vi "Get nidaqmx_grpc_GetChanAttributeStringRequest.vi"(8 "error in (no error)":errorcluster, 11 "gRPCid":T1) -> (0 "error out":errorcluster, 2 "package_templatemessage":T2, 3 "gRPCid out":T1)   [LabVIEW 2021, in "NI DAQmx_server.lvlib"]
uses:
  NI DAQmx_server.lvlib
  nidaqmx_grpc_GetChanAttributeStringRequest.ctl
  nidevice_grpc_Session_session/nidevice_grpc_Session_session.lvclass
  nidaqmx_grpc_GetChanAttributeStringRequest_attribute_enum/nidaqmx_grpc_GetChanAttributeStringRequest_attribute_enum.lvclass
  nidevice_grpc_Session.ctl
  <vilib>/gRPC/LabVIEW gRPC Library/Shared/grpcId.ctl
  nidaqmx_grpc_GetChanAttributeStringRequest_Flat.ctl
  nidevice_grpc_Session_Flat.ctl
  nidaqmx_grpc_ChannelStringAttribute.ctl
  nidevice_grpc_Session_session/nidevice_grpc_Session_session.lvclass/nidevice_grpc_Session_session.ctl
  nidaqmx_grpc_GetChanAttributeStringRequest_attribute_enum/nidaqmx_grpc_GetChanAttributeStringRequest_attribute_enum.lvclass/nidaqmx_grpc_GetChanAttributeStringRequest_attribute_enum.ctl
  2ed25e12-861d-4677-8ead-ace2906b2041.vi
  <vilib>/gRPC/LabVIEW gRPC Library/Shared/TranslateGrpcError.vi
  FlatToRichnidevice_grpc_Session.vi
  nidaqmx_grpc_GetChanAttributeStringRequest_attribute_enum/Setattribute.vi
  nidaqmx_grpc_GetChanAttributeStringRequest_attribute_enum/Setattribute_raw.vi
  nidevice_grpc_Session_session/Setname.vi
  nidevice_grpc_Session_session/Setid.vi
  <vilib>/gRPC/LabVIEW gRPC Library/Server API/Server/Get Server DLL Path.vi
  <vilib>/Utility/error.llb/Error Cluster From Error Code.vi
  nidaqmx_grpc_GetChanAttributeStringRequest_attribute_enum/GetFieldFromProtobufIndexnidaqmx_grpc_GetChanAttributeStringRequest_attribute_enum.vi
  nidevice_grpc_Session_session/GetFieldFromProtobufIndexnidevice_grpc_Session_session.vi
  <vilib>/gRPC/LabVIEW gRPC Library/grpc-lvsupport-release.lvlib
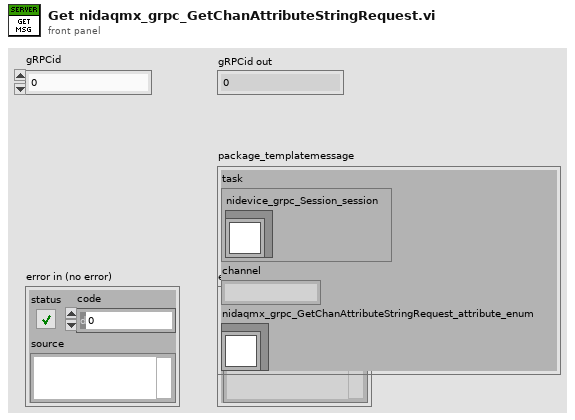
[diagram p1: front panel]
types:
  T1 = typedef "grpc-lvsupport-release.lvlib/grpcId.ctl" = u64
  T2 = typedef "NI DAQmx_server.lvlib/nidaqmx_grpc_GetChanAttributeStringRequest.ctl" = cluster{"task":T3, "channel":string, "nidaqmx_grpc_GetChanAttributeStringRequest_attribute_enum":refnum<class "nidaqmx_grpc_GetChanAttributeStringRequest_attribute_enum.lvclass">}
  T3 = typedef "NI DAQmx_server.lvlib/nidevice_grpc_Session.ctl" = cluster{"nidevice_grpc_Session_session":refnum<class "nidevice_grpc_Session_session.lvclass">}
  T4 = typedef "NI DAQmx_server.lvlib/nidaqmx_grpc_GetChanAttributeStringRequest_Flat.ctl" = cluster{"task":T5, "channel":string, "nidaqmx_grpc_GetChanAttributeStringRequest_attribute_enum_selected_index":i32, "attribute":T6, "attribute_raw":i32}
  T5 = typedef "NI DAQmx_server.lvlib/nidevice_grpc_Session_Flat.ctl" = cluster{"nidevice_grpc_Session_session_selected_index":i32, "name":string, "id":u32}
  T6 = typedef "NI DAQmx_server.lvlib/nidaqmx_grpc_ChannelStringAttribute.ctl" = enum32{"CHANNEL_STRING_ATTRIBUTE_UNSPECIFIED", "CHANNEL_ATTRIBUTE_CI_CTR_TIMEBASE_SRC", "CHANNEL_ATTRIBUTE_CO_CTR_TIMEBASE_SRC", "CHANNEL_ATTRIBUTE_AI_THRMCPL_CJC_CHAN", "CHANNEL_ATTRIBUTE_CI_GPS_SYNC_SRC", "CHANNEL_ATTRIBUTE_AO_CUSTOM_SCALE_NAME", "CHANNEL_ATTRIBUTE_AI_CUSTOM_SCALE_NAME", "CHANNEL_ATTRIBUTE_CI_CUSTOM_SCALE_NAME", "CHANNEL_ATTRIBUTE_CI_FREQ_TERM", "CHANNEL_ATTRIBUTE_CI_PERIOD_TERM", "CHANNEL_ATTRIBUTE_CI_PULSE_WIDTH_TERM", "CHANNEL_ATTRIBUTE_CI_TWO_EDGE_SEP_FIRST_TERM", "CHANNEL_ATTRIBUTE_CI_TWO_EDGE_SEP_SECOND_TERM", "CHANNEL_ATTRIBUTE_CI_SEMI_PERIOD_TERM", "CHANNEL_ATTRIBUTE_CI_COUNT_EDGES_TERM", "CHANNEL_ATTRIBUTE_CO_PULSE_TERM", "CHANNEL_ATTRIBUTE_PHYSICAL_CHAN_NAME", "CHANNEL_ATTRIBUTE_CHAN_DESCR", "CHANNEL_ATTRIBUTE_AI_INPUT_SRC", "CHANNEL_ATTRIBUTE_CI_ENCODER_A_INPUT_TERM", "CHANNEL_ATTRIBUTE_CI_ENCODER_B_INPUT_TERM", "CHANNEL_ATTRIBUTE_CI_ENCODER_Z_INPUT_TERM", "CHANNEL_ATTRIBUTE_AI_TEDS_UNITS", "CHANNEL_ATTRIBUTE_CI_COUNT_EDGES_DIR_TERM", "CHANNEL_ATTRIBUTE_CI_FREQ_DIG_FLTR_TIMEBASE_SRC", "CHANNEL_ATTRIBUTE_CI_PERIOD_DIG_FLTR_TIMEBASE_SRC", "CHANNEL_ATTRIBUTE_CI_COUNT_EDGES_COUNT_DIR_DIG_FLTR_TIMEBASE_SRC", "CHANNEL_ATTRIBUTE_CI_COUNT_EDGES_DIG_FLTR_TIMEBASE_SRC", "CHANNEL_ATTRIBUTE_CI_ENCODER_A_INPUT_DIG_FLTR_TIMEBASE_SRC", "CHANNEL_ATTRIBUTE_CI_ENCODER_B_INPUT_DIG_FLTR_TIMEBASE_SRC", "CHANNEL_ATTRIBUTE_CI_ENCODER_Z_INPUT_DIG_FLTR_TIMEBASE_SRC", "CHANNEL_ATTRIBUTE_CI_PULSE_WIDTH_DIG_FLTR_TIMEBASE_SRC", "CHANNEL_ATTRIBUTE_CI_TWO_EDGE_SEP_FIRST_DIG_FLTR_TIMEBASE_SRC", "CHANNEL_ATTRIBUTE_CI_TWO_EDGE_SEP_SECOND_DIG_FLTR_TIMEBASE_SRC", "CHANNEL_ATTRIBUTE_CI_SEMI_PERIOD_DIG_FLTR_TIMEBASE_SRC", "CHANNEL_ATTRIBUTE_AO_DAC_REF_EXT_SRC", "CHANNEL_ATTRIBUTE_AO_DAC_OFFSET_EXT_SRC", "CHANNEL_ATTRIBUTE_CI_CTR_TIMEBASE_DIG_FLTR_TIMEBASE_SRC", "CHANNEL_ATTRIBUTE_CO_CTR_TIMEBASE_DIG_FLTR_TIMEBASE_SRC", "CHANNEL_ATTRIBUTE_AI_CHAN_CAL_OPERATOR_NAME", "CHANNEL_ATTRIBUTE_AI_CHAN_CAL_DESC", "CHANNEL_ATTRIBUTE_DI_DIG_FLTR_TIMEBASE_SRC", "CHANNEL_ATTRIBUTE_CI_PULSE_FREQ_TERM", "CHANNEL_ATTRIBUTE_CI_PULSE_FREQ_DIG_FLTR_TIMEBASE_SRC", "CHANNEL_ATTRIBUTE_CI_PULSE_TIME_TERM", "CHANNEL_ATTRIBUTE_CI_PULSE_TIME_DIG_FLTR_TIMEBASE_SRC", "CHANNEL_ATTRIBUTE_CI_PULSE_TICKS_TERM", "CHANNEL_ATTRIBUTE_CI_PULSE_TICKS_DIG_FLTR_TIMEBASE_SRC", "CHANNEL_ATTRIBUTE_CI_COUNT_EDGES_COUNT_RESET_TERM", "CHANNEL_ATTRIBUTE_CI_COUNT_EDGES_COUNT_RESET_DIG_FLTR_TIMEBASE_SRC", "CHANNEL_ATTRIBUTE_AI_ROSETTE_STRAIN_GAGE_STRAIN_CHANS", "CHANNEL_ATTRIBUTE_CI_TIMESTAMP_TERM", "CHANNEL_ATTRIBUTE_NAV_CUSTOM_SCALE_NAME", "CHANNEL_ATTRIBUTE_CI_DUTY_CYCLE_TERM", "CHANNEL_ATTRIBUTE_CI_DUTY_CYCLE_DIG_FLTR_TIMEBASE_SRC", "CHANNEL_ATTRIBUTE_CI_VELOCITY_ENCODER_A_INPUT_TERM", "CHANNEL_ATTRIBUTE_CI_VELOCITY_ENCODER_A_INPUT_DIG_FLTR_TIMEBASE_SRC", "CHANNEL_ATTRIBUTE_CI_VELOCITY_ENCODER_B_INPUT_TERM", "CHANNEL_ATTRIBUTE_CI_VELOCITY_ENCODER_B_INPUT_DIG_FLTR_TIMEBASE_SRC", "CHANNEL_ATTRIBUTE_CI_COUNT_EDGES_GATE_TERM", "CHANNEL_ATTRIBUTE_CI_COUNT_EDGES_GATE_DIG_FLTR_TIMEBASE_SRC"}
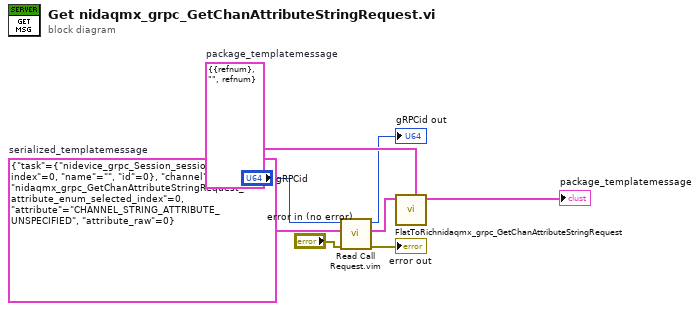
[diagram p0: block diagram]
diagram:
  w6 = T4 {"task"={"nidevice_grpc_Session_session_selected_index"=0, "name"="", "id"=0}, "channel"="", "nidaqmx_grpc_GetChanAttributeStringRequest_attribute_enum_selected_index"=0, "attribute"=enum."CHANNEL_STRING_ATTRIBUTE_UNSPECIFIED", "attribute_raw"=0}  # serialized_templatemessage
  w5 = T2 {"task"={"nidevice_grpc_Session_session"=refnum}, "channel"="", "nidaqmx_grpc_GetChanAttributeStringRequest_attribute_enum"=refnum}  # package_templatemessage
  n1 = call "Read Call Request.vim"("error in"="error in (no error)", "Request Type"=w6, "gRPCid in"="gRPCid") -> ("error out"=→"error out":errorcluster, "Request Data"=w4:T4, "gRPCid out"=→"gRPCid out":T1)  [unwired: 6 in]
  n2 = call "FlatToRichnidaqmx_grpc_GetChanAttributeStringRequest.vi"("OutputClusterType"=w5, "InputCluster"=w4) -> ("OutputCluster"=→"package_templatemessage":T2)  [unwired: 9 in]
